vi "Set_PS2_16V.vi"(3 "error in":errorcluster) -> (10 "error out":errorcluster)   [LabVIEW 2015]
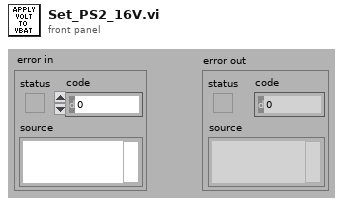
[diagram p1: front panel]
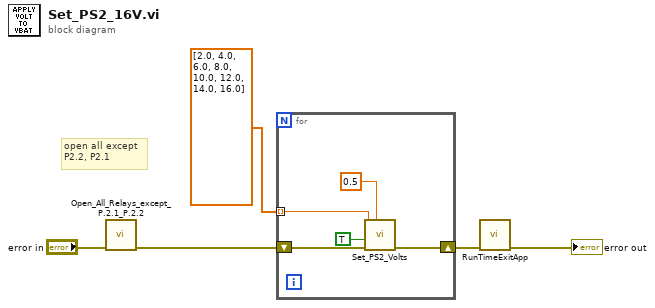
[diagram p0: block diagram]
diagram:
  # "open all except \nP2.2, P2.1"
  n1 = call "Open_All_Relays_except_P.2.1_P.2.2.vi"("error in"="error in") -> ("error out"=w3:errorcluster)  [unwired: 9 in]
  n2 = for {
    shift-right: [w9] -> w2
    shift-left: w3 -> [w10]
    tunnel: dbl[] [2.0, 4.0, 6.0, 8.0, 10.0, 12.0, 14.0, 16.0] -> [w6] mode=indexing
    n3 = call "Set_PS2_Volts.vi"("delay (secs)"=0.5, "error in"=w10, "Output on/off"=TRUE, "Output Voltage"=w6) -> ("error out"=w9:errorcluster)  [unwired: 5 in, 2 out]
  }
  n4 = call "RunTimeExitApp.vi"("error in (no error)"=w2) -> ("error out"=→"error out":errorcluster)  [unwired: 10 in]
